vi "Write.vi"(8 "error in (no error)":errorcluster, 10 "Write Buffer":string, 11 "VISA resource name":refnum<visa-resource-name>) -> (0 "error out":errorcluster, 3 "VISA resource name out":refnum<visa-resource-name>)   [LabVIEW 2015, in "Voltech PM1000+.lvlib"]
doc: "Writes semicolon (;) seperated IEEE 488.2 compatible commands into instrument. \nSeparates command string (ex. :SEL:VLT;:SEL:AMP;:SEL:WAT) into several single command (ex. :SEL:VLT, :SEL:AMP, :SEL:WAT) and sends them to the instrument."
uses:
  <instrlib>/Voltech PM1000+/Voltech PM1000+.lvlib
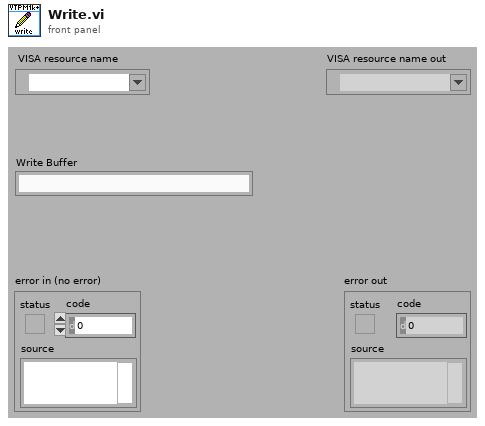
[diagram p1: front panel]
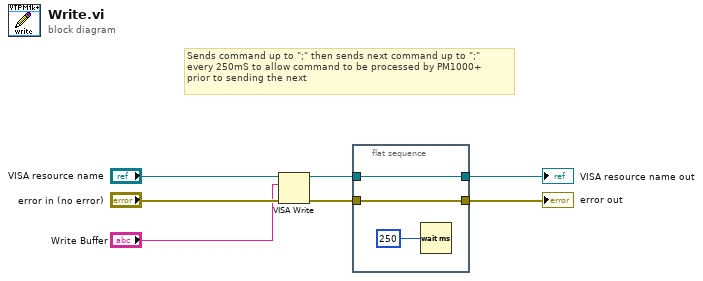
[diagram p0: block diagram]
diagram:
  # "Sends command up to \";\" then sends next command up to \";\"\nevery 250mS to allow command to be processed by PM1000+\nprior to sending the next"
  n1 = VISA Write(VISA resource name="VISA resource name", write buffer="Write Buffer", error in (no error)="error in (no error)") -> (VISA resource name out=w5:refnum<visa-resource-name>, error out=w4:errorcluster)  [unwired: 1 out]
  n2 = flat-sequence {
    tunnel: [w9] -> w2
    tunnel: w5 -> [w9]
    tunnel: [w8] -> w3
    tunnel: w4 -> [w8]
    frame #0 {
      n3 = Wait (ms)(milliseconds to wait=250) -> ()  [unwired: 1 out]
    }
  }
  "error out" <- w3
  "VISA resource name out" <- w2
